vi "InitLayoutRing.vi"(7 "Layouts Ring Refnum":refnum<vi>, 8 "error in (no error)":errorcluster) -> (0 "error out":errorcluster)   [LabVIEW 2013]
uses:
  <vilib>/Utility/miscctls.llb/LVStringsAndValuesArrayTypeDef_I32.ctl
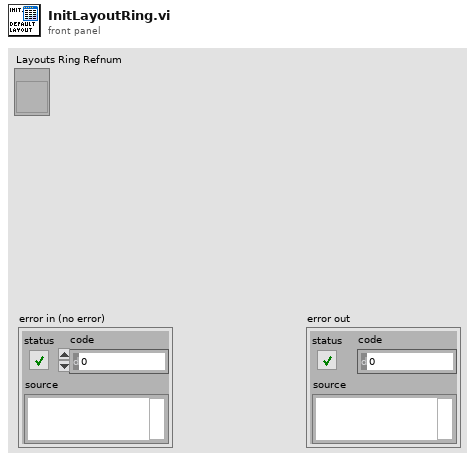
[diagram p1: front panel]
types:
  T1 = typedef "LVStringsAndValuesArrayTypeDef_I32.ctl" = cluster{"String":string, "Value":i32}[]
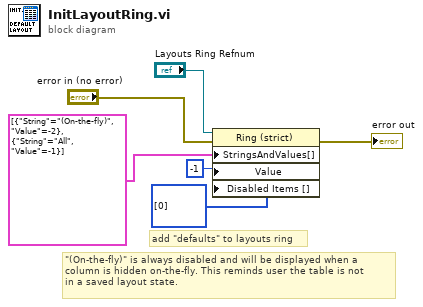
[diagram p0: block diagram]
diagram:
  # "\"(On-the-fly)\" is always disabled and will be displayed when a \ncolumn is hidden on-the-fly. This reminds user the table is not\nin a saved layout state."
  # "add \"defaults\" to layouts ring"
  n1 = property class="Ring (strict)"(reference="Layouts Ring Refnum", error in="error in (no error)", "StringsAndValues[]"=T1 [{"String"="(On-the-fly)", "Value"=-2}, {"String"="All", "Value"=-1}] ("Strings And Values []"), "Value"=-1, "Disabled Items []"=i32[] [0]) -> (error out=→"error out":errorcluster)  [unwired: 1 out]
